vi "align_angle.vi"(9 "Max Speed":dbl=3.0, 11 "Initial X, Y, BEARING":cluster{dbl, dbl, dbl}) -> (3 "Final X, Y, BEARING":cluster{dbl, dbl, dbl}={-30.068060606349714, 7954.135185370846, 4.207864617948657})   [LabVIEW 2017]
uses:
  <vilib>/myRIO/Common/Instrument Driver Framework/myRIO v1.0/Encoder/typedefs/Encoder Signal Mode.ctl
  <vilib>/myRIO/Instrument Drivers/Onboard IO/Encoder/typedefs/Encoder Reference.ctl
  <vilib>/myRIO/Common/Instrument Driver Framework/Utilities/typedefs/myRIO Generic Hardware Reference.ctl
  <vilib>/myRIO/Common/Instrument Driver Framework/Utilities/typedefs/Hardware Version Enum.ctl
  <vilib>/myRIO/Common/Instrument Driver Framework/Utilities/typedefs/myRIO v1.0 Reference.ctl
  <vilib>/myRIO/Common/Instrument Driver Framework/Utilities/typedefs/Generic FPGA Reference.ctl
  <vilib>/myRIO/Common/Instrument Driver Framework/myRIO v1.0/Encoder/typedefs/Encoder Channels Enum.ctl
  <vilib>/myRIO/Common/Instrument Driver Framework/myRIO v1.0/Encoder/typedefs/Encoder Configuration v1.0.ctl
  <vilib>/userdefined/High Color/nirio_resource_hc.ctl
  <vilib>/myRIO/Common/Instrument Driver Framework/Utilities/vis/Is FPGA Ref Available.vi
  <vilib>/myRIO/Common/Instrument Driver Framework/myRIO v1.0/Encoder/vis/myRIO v1.1 Open Encoder.vi
  <vilib>/myRIO/Instrument Drivers/Onboard IO/Encoder/vis/Read.vi
  <vilib>/myRIO/Common/Instrument Driver Framework/Utilities/vis/Validate Channels.vi
  <vilib>/myRIO/Common/Instrument Driver Framework/myRIO v1.0/Encoder/vis/myRIO v1.0 Reserve Encoder.vi
  <vilib>/myRIO/Common/Instrument Driver Framework/myRIO v1.0/Encoder/vis/myRIO v1.0 Build MUX Configuration Encoder.vi
  <vilib>/myRIO/Common/Instrument Driver Framework/myRIO v1.0/Resource Manager/vis/myRIO v1.0 Reserve Channel List.vi
  <vilib>/myRIO/Common/Instrument Driver Framework/myRIO v1.0/Resource Manager/vis/myRIO v1.0 Create Configuration List.vi
  <vilib>/myRIO/Common/Instrument Driver Framework/myRIO v1.0/Resource Manager/vis/myRIO v1.0 Reserve Channel.vi
  <vilib>/myRIO/Common/Instrument Driver Framework/myRIO v1.0/Resource Manager/vis/myRIO v1.0 Unreserve Channel.vi
  <vilib>/myRIO/Common/Instrument Driver Framework/myRIO v1.0/Resource Manager/vis/myRIO v1.0 Build Mutex Name.vi
  <vilib>/Utility/VariantDataType/GetNumericInfo.vi
  <vilib>/Utility/error.llb/Error Cluster From Error Code.vi
  <vilib>/myRIO/Common/Instrument Driver Framework/myRIO v1.0/myRIO v1.1 Open.vi
  <vilib>/myRIO/Common/Instrument Driver Framework/Utilities/vis/IO Manager.vi
  <vilib>/myRIO/Common/Instrument Driver Framework/Utilities/vis/Configuration Manager.vi
  <vilib>/myRIO/Common/Instrument Driver Framework/myRIO v1.0/Resource Manager/vis/myRIO v1.0 Configure IO.vi
  <vilib>/myRIO/Common/Instrument Driver Framework/myRIO v1.0/myRIO v1.0 Close.vi
  <vilib>/myRIO/Common/Instrument Driver Framework/myRIO v1.0/Encoder/vis/myRIO v1.0 Configure Encoder.vi
  <vilib>/myRIO/Common/Instrument Driver Framework/myRIO v1.0/Encoder/vis/myRIO v1.0 Read Encoder.vi
  <vilib>/addons/control/pid/pid.llb/PID (DBL).vi
  <vilib>/myRIO/Express VI/Onboard IO/Encoder/Encoder Express VI.xnode
  <vilib>/myRIO/Instrument Drivers/Onboard IO/Encoder/vis/myRIO Encoder Open.xnode
  <vilib>/myRIO/Common/Instrument Driver Framework/myRIO v1.0/Encoder/typedefs/Encoder Count Direction Enum.ctl
  <vilib>/addons/control/pid/NI_PID_pid.lvlib
  <vilib>/myRIO/Instrument Drivers/Onboard IO/Encoder/Encoder.lvlib
panel:
  out "Waveform Chart":dbl(graph)=4.207864617948657
  in  "angle":dbl(slide) scale=-90.0..90.0
  in  "speed":dbl(slide)=1.8691588785046729 scale=0.0..10.0
  in  "Min Speed":dbl=1.0
  out "XY Graph":cluster{"X":dbl, "Y":dbl}[](graph)=[{"X"=-30.082698286482174, "Y"=7953.93623198267}, {"X"=-30.068060606349714, "Y"=7954.135185370846}]
  in  "PID gains":T1={"proportional gain (Kc)"=0.04, "integral time (Ti, min)"=0.1, "derivative time (Td, min)"=0.0} {"derivative time (Td, min)" format="%.3f"; "integral time (Ti, min)" format="%.3f"; "proportional gain (Kc)" format="%.3f"}
  in  "stop":bool=TRUE
  out "OUTPUT B":dbl(slide)=3.0 scale=-10.0..10.0
  out "OUTPUT A":dbl(slide)=0.9259999999994761 scale=-10.0..10.0
  out "PID A":T2(graph)={"Setpoint"=1.7890362814617413, "output"=0.16204700765601243, "dx/dt"=0.9259999999994761}
  out "PID B":T2(graph)={"Setpoint"=1.9492814755476044, "output"=0.04903176938944572, "dx/dt"=3.0}
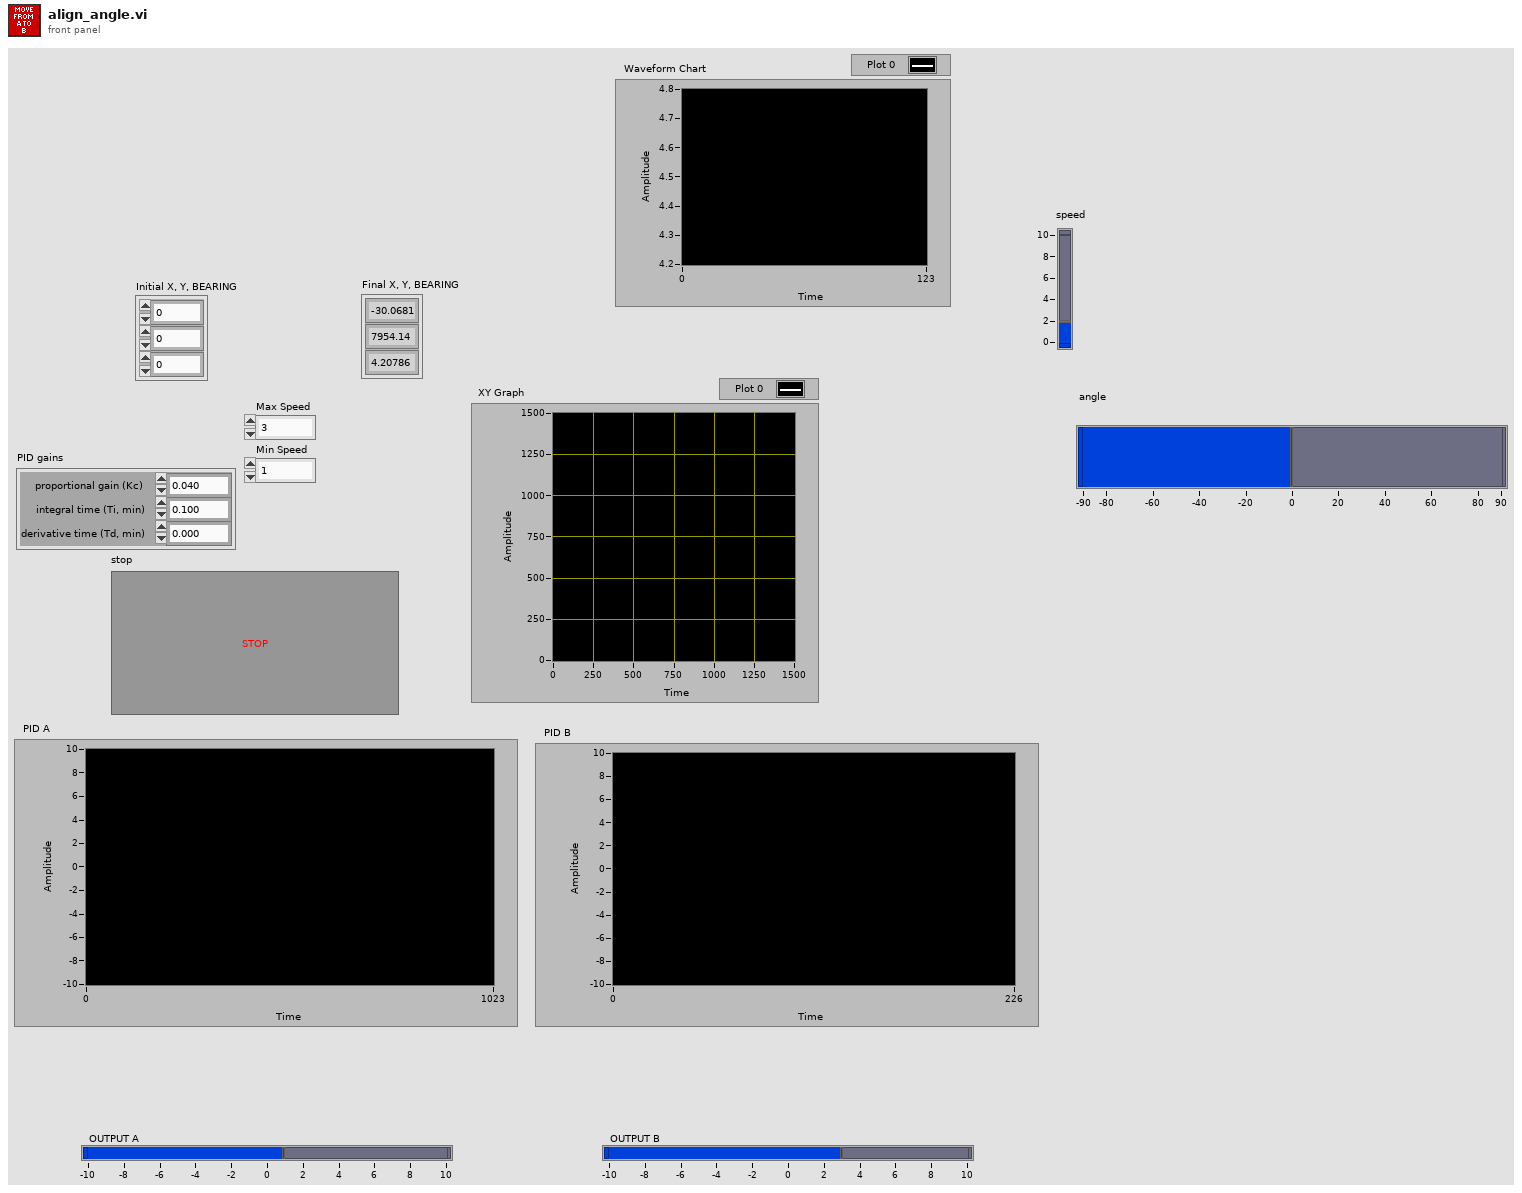
[diagram p1: front panel]
types:
  T1 = cluster{"proportional gain (Kc)":dbl, "integral time (Ti, min)":dbl, "derivative time (Td, min)":dbl}
  T2 = cluster{"Setpoint":dbl, "output":dbl, "dx/dt":dbl}
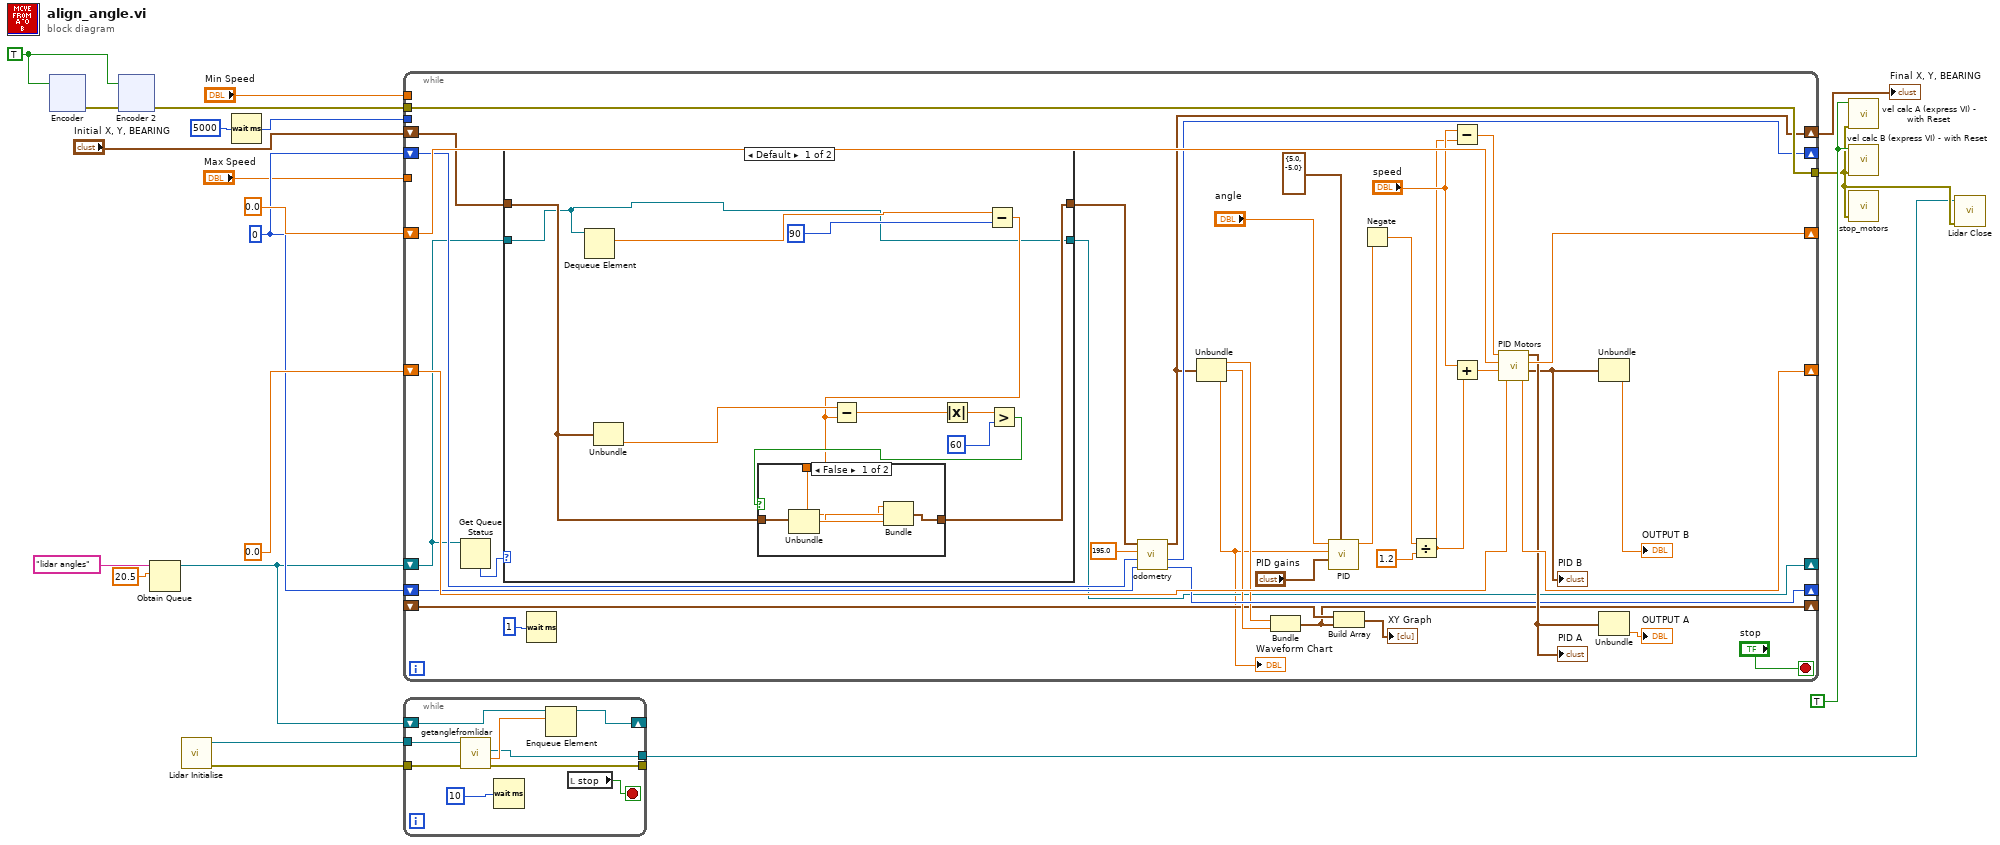
[diagram p0: block diagram]
diagram:
  w8 = TRUE ("Reinitialise")
  w10 = TRUE
  w14 = 0 ("ENCA OUT")
  n1 = xnode "Encoder"("Reset Counter"=w10) -> ("error out"=w11:errorcluster)  [unwired: 1 in, 3 out]
  n2 = xnode "Encoder 2"("error in (no error)"=w11, "Reset Counter"=w10) -> ("error out"=w9:errorcluster)  [unwired: 3 out]
  n3 = Obtain Queue(name (unnamed)="lidar angles", element data type=20.5) -> (queue out=w4:refnum<queue>)  [unwired: 3 in, 2 out]
  n4 = call "Lidar Initialise.vi"() -> ("error out"=w1:errorcluster, "VISA resource name out"=w7:refnum<visa-resource-name>)  [unwired: 10 in]
  n5 = Wait (ms)(milliseconds to wait=u32 5000) -> (millisecond timer value=w18:u32)
  n6 = while {
    tunnel: w9 -> [w52]
    shift-right: [w54] -> _
    shift-left: 0.0 ("output A") -> [w55]
    shift-right: [w57] -> _
    shift-left: 0.0 ("output B") -> [w56]
    tunnel: [w52] -> w3
    shift-right: [w44] -> _
    shift-left: w14 -> [w46]
    shift-right: [w43] -> _
    shift-left: w14 -> [w45]
    shift-right: [w30] -> w20
    shift-left: "Initial X, Y, BEARING" -> [w34]
    shift-right: [w39] -> _
    shift-left: _ -> [w40]
    tunnel: "Max Speed" -> [_]
    tunnel: "Min Speed" -> [_]
    tunnel: w18 -> [_]
    shift-right: [w31] -> _
    shift-left: w4 -> [w32]
    stop <- "stop" stop-if-true
    n7 = Get Queue Status(queue=w32) -> (# elements in queue=w35:i32)  [unwired: 2 in, 7 out]
    n8 = case shown="Default" w35 {
      tunnel: w34 -> [w63 w77]
      tunnel: [w64 w77] -> w33
      tunnel: w32 -> [w59 w76]
      tunnel: [w59 w76] -> w31
      frame Default {
        n9 = Dequeue Element(queue=w59) -> (element=w60:dbl)  [unwired: 2 in, 3 out]
        n10 = Unbundle(w63) -> (w62:dbl)  [unwired: 2 out]
        n11 = Subtract(x=w60, y=90) -> (x-y=w61:dbl)
        n12 = Subtract(x=w62, y=w61) -> (x-y=w68:dbl)
        n13 = Absolute Value(x=w68) -> (abs(x)=w67:dbl)
        n14 = Greater?(x=w67, y=60) -> (0:w65:bool)
        n15 = case shown="False" w65 {
          tunnel: w63 -> [w74 w75]
          tunnel: [w70 w75] -> w64
          tunnel: w61 -> [w73 _]
          frame False {
            n16 = Unbundle(w74) -> (w71:dbl, w72:dbl)  [unwired: 1 out]
            n17 = Bundle(w71, w72, w73) -> (w70:cluster{dbl, dbl, dbl})  [unwired: 1 in]
          }
          frame True {
          }
        }
      }
      frame 0 {
      }
    }
    n18 = Wait (ms)(milliseconds to wait=1 ("ENCB OUT")) -> ()  [unwired: 1 out]
    n19 = call "odometry.vi"("ENCB in"=w45, "ENCA in"=w46, "wheelbase"=195.0, "Position"=w33) -> ("ENCB OUT"=w43:i32, "ENCA OUT"=w44:i32, "X, Y, BEARING"=w30:cluster{dbl, dbl, dbl})  [unwired: 4 in]
    n20 = Unbundle(w30) -> (w41:dbl, w42:dbl, w25:dbl)
    "Waveform Chart" <- w25
    n21 = Bundle(w41, w42) -> (w39:cluster{dbl, dbl})  [unwired: 1 in]
    n22 = call-poly <vilib>:"PID.vi"("output range"=cluster{"output high":dbl, "output low":dbl} {"output high"=5.0, "output low"=-5.0}, "PID gains"="PID gains", "process variable"=w25, "setpoint"="angle") -> ("output"=w22:dbl)  [unwired: 6 in, 1 out]
    n23 = Build Array(w40, w39) -> (→"XY Graph":cluster{dbl, dbl}[])
    n24 = Negate(x=w22) -> (-x=w21:dbl)
    n25 = Divide(x=w21, y=1.2) -> (x/y=w24:dbl)
    n26 = Subtract(x="speed", y=w24) -> (x-y=w27:dbl)
    n27 = Add(x="speed", y=w24) -> (x+y=w26:dbl)
    n28 = call "PID Motors.vi"("input B"=w56, "Speed B"=w26, "input A"=w55, "Speed A"=w27) -> ("output B"=w57:dbl, "Speed B0"=w50:T2, "output A"=w54:dbl, "Speed A0"=w51:T2)
    "PID B" <- w50
    "PID A" <- w51
    n29 = Unbundle(w50) -> ("dx/dt"=→"OUTPUT B":dbl)  [unwired: 2 out]
    n30 = Unbundle(w51) -> ("dx/dt"=→"OUTPUT A":dbl)  [unwired: 2 out]
  }
  "Final X, Y, BEARING" <- w20
  n31 = while {
    tunnel: w7 -> [w86]
    shift-right: [w82] -> _
    shift-left: w4 -> [w84]
    tunnel: [w81] -> w2
    tunnel: w1 -> [w80]
    tunnel: [w79] -> _
    stop <- w85 stop-if-true
    n32 = call "getanglefromlidar.vi"("error in (no error)"=w80, "VISA resource name"=w86) -> ("error constant"=w79:errorcluster, "Angle From WALL"=w83:dbl, "VISA resource name out"=w81:refnum<visa-resource-name>)  [unwired: 4 in, 3 out]
    n33 = Wait (ms)(milliseconds to wait=10 ("ENCB OUT")) -> ()  [unwired: 1 out]
    n34 = Enqueue Element(queue=w84, element=w83) -> (queue out=w82:refnum<queue>)  [unwired: 2 in, 2 out]
    n35 = local read "stop"() -> (w85:bool)
  }
  n36 = call "vel calc A (express VI) - with Reset.vi"("error in"=w3, "Reinitialise"=w8) -> ()  [unwired: 5 in, 5 out]
  n37 = call "vel calc B (express VI) - with Reset.vi"("error in"=w3, "Reinitialise"=w8) -> ()  [unwired: 5 in, 5 out]
  n38 = call "stop_motors.vi"("error in (no error)"=w3) -> ()  [unwired: 4 in, 1 out]
  n39 = call "Lidar Close.vi"("error in (no error)"=w3, "VISA resource name"=w2) -> ()  [unwired: 9 in, 1 out]
